vi "getStatus.vi"(8 "error in (no error)":errorcluster, 11 "DDSOutput in":refnum<class "DDSOutput.lvclass">) -> (0 "error out":errorcluster, 2 "status array":bool[](array[boolean]), 3 "DDSOutput out":refnum<class "DDSOutput.lvclass">)   [LabVIEW 2009, in "Hardware.lvlib" / "Channels.lvlib" / "DDSOutput.lvclass"]
uses:
  DDSOutput.lvclass
panel:
  # "SpinCore Status:\n\npb_read_status(void) returns a 32 bit int:\nbit0 :stopped\nbit1: Reset\nbit2:Running\nbit3: Waiting\nBit4: Scanning (not this board)\nBit5-31 are reserved for future use.\n\nSee SpinAPI reference for details"
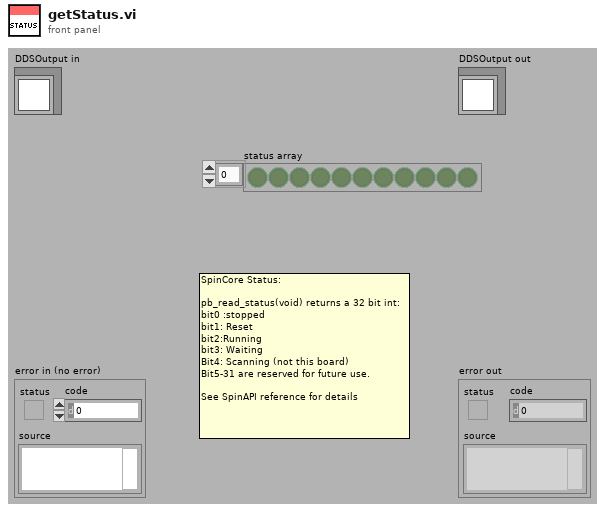
[diagram p1: front panel]
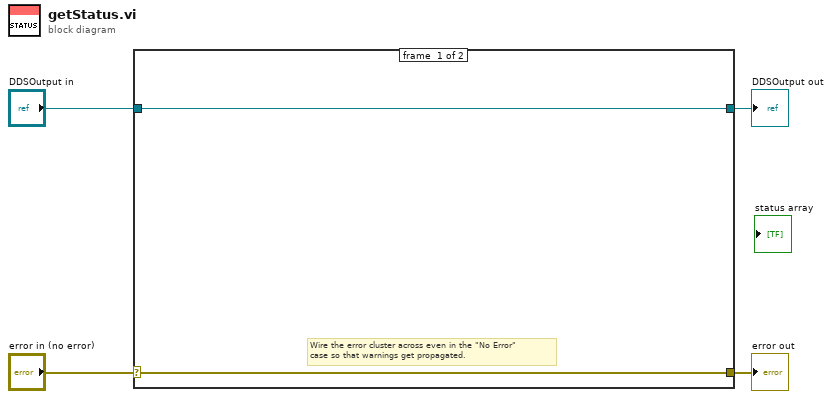
[diagram p0: block diagram]
diagram:
  n1 = case shown="No Error" "error in (no error)" {
    selector: "error in (no error)" -> [w5 w8]
    tunnel: [w5 w8] -> w3
    tunnel: [w6 w7] -> w1
    tunnel: "DDSOutput in" -> [w6 w7]
    frame #0 {
      # "Wire the error cluster across even in the \"No Error\"\ncase so that warnings get propagated."
    }
    frame #1 {
    }
  }
  "error out" <- w3
  "DDSOutput out" <- w1
